vi "GCMPlugin_IsSupportingItem.vi"(8 "error in (no error)":errorcluster, 9 "VI Reference":refnum<vi>, 10 "ProjectItem Refnum":refnum<vi>, 11 "TemplatePlugin in":refnum<class "InstallerSpecEditor.lvclass">) -> (0 "error out":errorcluster, 2 "IsSupportingItem":bool, 3 "TemplatePlugin out":refnum<class "InstallerSpecEditor.lvclass">)   [LabVIEW 2014, in "BuildSpecEditor.lvlib" / "InstallerSpecEditor.lvclass"]
uses:
  InstallerSpecEditor.lvclass
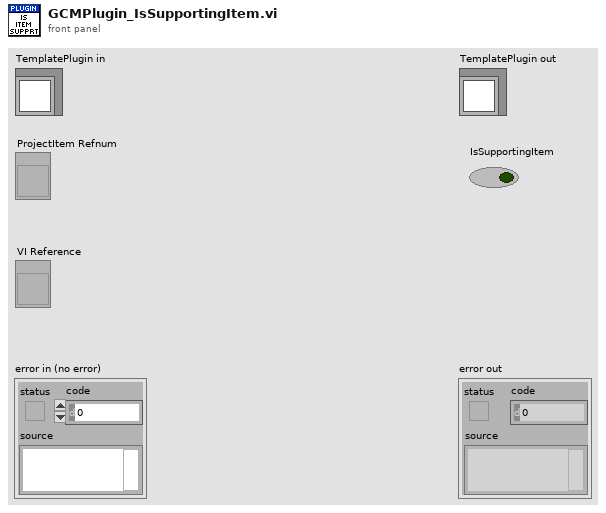
[diagram p1: front panel]
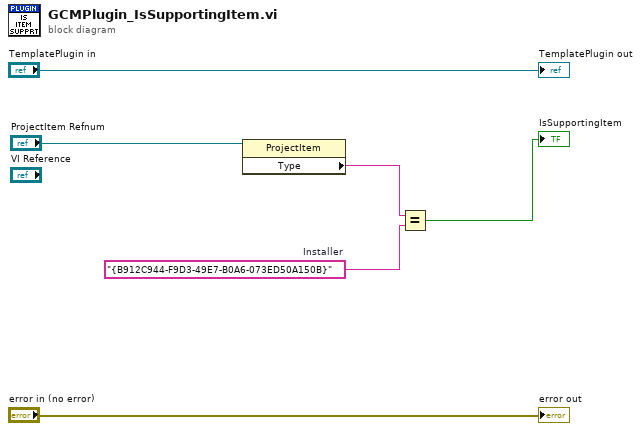
[diagram p0: block diagram]
diagram:
  w2 = "{B912C944-F9D3-49E7-B0A6-073ED50A150B}"  # Installer
  n1 = property class="ProjectItem"(reference="ProjectItem Refnum") -> ("Type"=w3:string)  [unwired: 1 in, 2 out]
  n2 = Equal?(x=w3, y=w2) -> (x = y?=→"IsSupportingItem":bool)
  "error out" <- "error in (no error)"
  "TemplatePlugin out" <- "TemplatePlugin in"
